vi "To I2C Data Packet.vi"(4 "Color Number":u8, 6 "Manual Color":bool, 9 "Section":u8, 10 "Pattern":T2=enum."Solid", 11 "Color":T1) -> (1 "Output Byte 3":u8, 2 "Output Byte 2":u8, 3 "Output Byte":u8)   [LabVIEW 2014]
doc: "This VI takes the configuration input and gives you the packet to send to the Arduino."
uses:
  LED_Patterns.ctl
  LED_Colors.ctl
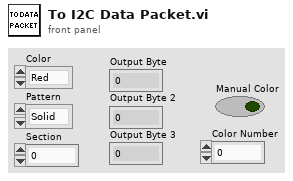
[diagram p1: front panel]
types:
  T1 = typedef "LED_Colors.ctl" = enum8{"Red", "Green", "Blue", "Cyan", "Magenta", "Yellow"}
  T2 = typedef "LED_Patterns.ctl" = enum8{"Black White", "Solid", "Blink", "Sweep", "Sleep"}
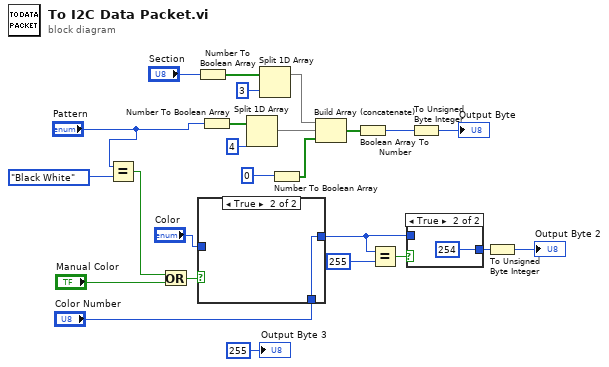
[diagram p0: block diagram]
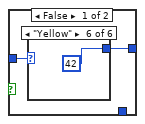
[diagram p2: hidden frame]
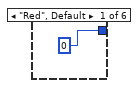
[diagram p3: hidden frame]
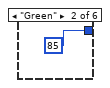
[diagram p4: hidden frame]
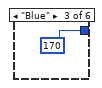
[diagram p5: hidden frame]
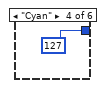
[diagram p6: hidden frame]
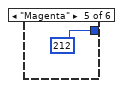
[diagram p7: hidden frame]
diagram:
  n1 = Equal?(x="Pattern", y=LED_Patterns."Black White" ("Pattern 2")) -> (x = y?=w3:bool)
  n2 = Or(x=w3, y="Manual Color") -> (x .or. y?=w4:bool)
  n3 = Number To Boolean Array(number="Section") -> (Boolean array=w23:bool[])
  n4 = case shown="True" w4 {
    tunnel: "Color" -> [w27 _]
    tunnel: [w26 w34] -> w7
    tunnel: "Color Number" -> [_ w34]
    frame False {
      n5 = case shown="\"Yellow\"" w27 {
        tunnel: [0 85 170 127 212 42] -> w26
        frame "Red", Default {
        }
        frame "Green" {
        }
        frame "Blue" {
        }
        frame "Cyan" {
        }
        frame "Magenta" {
        }
        frame "Yellow" {
        }
      }
    }
    frame True {
    }
  }
  n6 = Number To Boolean Array(number="Pattern") -> (Boolean array=w24:bool[])
  n7 = Split 1D Array(array=w24, index=4) -> (first subarray=w15:bool[])  [unwired: 1 out]
  n8 = Split 1D Array(array=w23, index=3) -> (first subarray=w16:bool[])  [unwired: 1 out]
  n9 = Number To Boolean Array(number=0) -> (Boolean array=w14:bool[])
  n10 = Build Array (concatenate)(w16, w15, w14) -> (w20:bool[])
  n11 = Boolean Array To Number(Boolean array=w20) -> (number=w19:u32)
  n12 = Equal?(x=w7, y=u8 255) -> (x = y?=w11:bool)
  n13 = case shown="True" w11 {
    tunnel: [w35 254] -> w10
    tunnel: w7 -> [w35 _]
    frame False {
    }
    frame True {
    }
  }
  n14 = To Unsigned Byte Integer(number=w19) -> (unsigned 8bit integer=→"Output Byte":u8)
  n15 = To Unsigned Byte Integer(number=w10) -> (unsigned 8bit integer=→"Output Byte 2":u8)
  "Output Byte 3" <- u8 255 ("Output Byte 3")
